vi "ZigZag galvo mirror module.vi"() -> ()   [LabVIEW 2025]
uses:
  <vilib>/DAQmx/write.llb/DAQmx Write (Analog 1D Wfm NChan NSamp).vi
  <vilib>/DAQmx/create/channels.llb/DAQmx Create Channel (AO-Voltage-Basic).vi
  <vilib>/DAQmx/configure/timing.llb/DAQmx Timing (Sample Clock).vi
  <vilib>/DAQmx/miscellaneous.llb/DAQmx Fill In Error Info.vi
  <vilib>/Analysis/1siggen.llb/Ramp Pattern by Samples.vi
  <vilib>/Analysis/NI_AALBase.lvlib
panel:
  out "appended array 2":waveform(dbl)[](array[waveform])
  out "appended array":dbl[][](array[numeric])
  in  "sample mode":i32(ring)=10178 items=["Finite Samples"=10178, "Continuous Samples"=10123, "Hardware Timed Single Point"=12522]
  in  "String":string
  in  "Pixel Rate (Hz)":dbl
  in  "Max Voltage (V)":dbl
  in  "Min Voltage (V)":dbl
  in  "Lines per frame (Y)":dbl
  in  "Pixel per line (X)":dbl
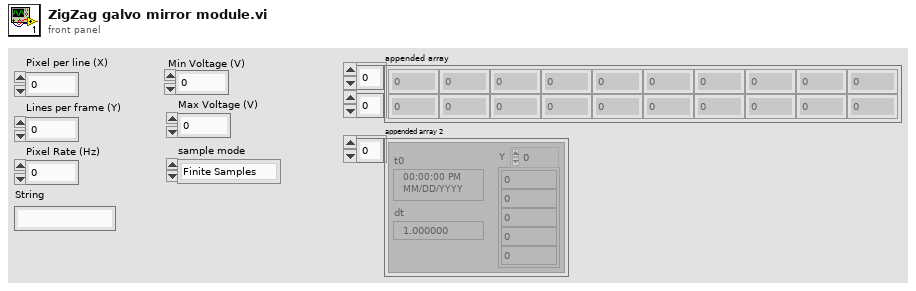
[diagram p1: front panel]
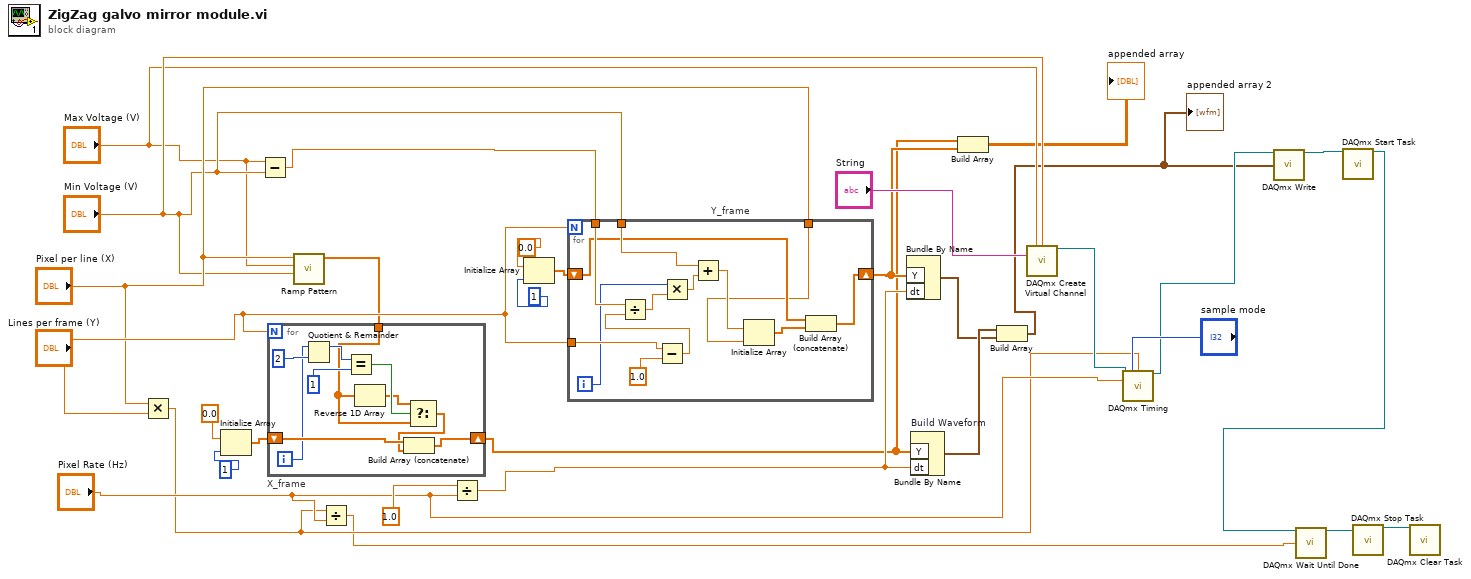
[diagram p0: block diagram]
diagram:
  n1 = Multiply(x="Pixel per line (X)", y="Lines per frame (Y)") -> (x*y=w6:dbl)
  n2 = Initialize Array(0.0 ("element"), 1 ("dimension size")) -> (w17:dbl[])
  n3 = Subtract(x="Max Voltage (V)", y="Min Voltage (V)") -> (x-y=w16:dbl)
  n4 = call-poly <vilib>:"Ramp Pattern.vi"("start"="Min Voltage (V)", "end"="Max Voltage (V)", "samples"="Pixel per line (X)") -> ("Ramp Pattern"=w12:dbl[])  [unwired: 7 in, 1 out]
  n5 = for "X_frame" {
    N: "Lines per frame (Y)" -> [_]
    shift-right: [w40] -> w9
    shift-left: w17 -> [w41]
    tunnel: w12 -> [w34]
    i -> [w35]
    n6 = Quotient & Remainder(x=w35, y=2) -> (x-y*floor(x/y)=w38:i32)  [unwired: 1 out]
    n7 = Equal?(x=w38, y=1) -> (x = y?=w36:bool)
    n8 = Reverse 1D Array(array=w34) -> (reversed array=w33:dbl[])
    n9 = Select(t=w33, s=w36, f=w34) -> (s? t:f=w32:dbl[])
    n10 = Build Array (concatenate)(w41, w32) -> (w40:dbl[])
  }
  n11 = Divide(x=w6, y="Pixel Rate (Hz)") -> (x/y=w5:dbl)
  n12 = Divide(x=1.0, y="Pixel Rate (Hz)") -> (x/y=w25:dbl)
  n13 = Initialize Array(0.0 ("element"), 1 ("dimension size")) -> (w30:dbl[])
  n14 = for "Y_frame" {
    N: "Lines per frame (Y)" -> [_]
    tunnel: "Lines per frame (Y)" -> [w54]
    tunnel: w16 -> [w52]
    tunnel: "Min Voltage (V)" -> [w47]
    tunnel: "Pixel per line (X)" -> [w42]
    shift-right: [w43] -> w10
    shift-left: w30 -> [w44]
    i -> [w49]
    n15 = Subtract(x=w54, y=1.0) -> (x-y=w51:dbl)
    n16 = Divide(x=w52, y=w51) -> (x/y=w50:dbl)
    n17 = Multiply(x=w49, y=w50) -> (x*y=w48:dbl)
    n18 = Add(x=w47, y=w48) -> (x+y=w46:dbl)
    n19 = Initialize Array "Initialize Array"(w46, w42) -> (w45:dbl[])
    n20 = Build Array (concatenate)(w44, w45) -> (w43:dbl[])
  }
  n21 = Bundle By Name("Y"=w10, "dt"=w25) -> (w23:waveform(dbl))  [unwired: 1 in]
  n22 = Bundle By Name "Build Waveform"("Y"=w9, "dt"=w25) -> (w24:waveform(dbl))  [unwired: 1 in]
  n23 = Build Array(w9, w10) -> (→"appended array":dbl[][])
  n24 = Build Array(w24, w23) -> (w1:waveform(dbl)[])
  "appended array 2" <- w1
  n25 = call-poly <vilib>:"DAQmx Create Virtual Channel.vi"("maximum value"="Max Voltage (V)", "minimum value"="Min Voltage (V)", "physical channels"="String") -> ("task out"=w20:refnum<k21>)  [unwired: 11 in, 1 out]
  n26 = call-poly <vilib>:"DAQmx Timing.vi"("task/channels in"=w20, "sample mode"="sample mode", "samples per channel"=w6, "rate"="Pixel Rate (Hz)") -> ("task out"=w11:refnum<k21>)  [unwired: 10 in, 1 out]
  n27 = call-poly <vilib>:"DAQmx Write.vi"("task/channels in"=w11, "data"=w1) -> ("task out"=w19:refnum<k21>)  [unwired: 11 in, 2 out]
  n28 = call <vilib>:"DAQmx Start Task.vi"("task/channels in"=w19) -> ("task out"=w4:refnum<k21>)  [unwired: 13 in, 1 out]
  n29 = call <vilib>:"DAQmx Wait Until Done.vi"("task/channels in"=w4, "timeout (sec)"=w5) -> ("task out"=w2:refnum<k21>)  [unwired: 12 in, 1 out]
  n30 = call <vilib>:"DAQmx Stop Task.vi"("task/channels in"=w2) -> ("task out"=w3:refnum<k21>)  [unwired: 13 in, 1 out]
  n31 = call <vilib>:"DAQmx Clear Task.vi"("task in"=w3) -> ()  [unwired: 14 in, 1 out]
